vi "Substitute the assigned name for BuildSpecification.vi"(8 "error in":errorcluster, 11 "PluginGenerator_MetaDataObj":refnum<class "PluginGenerator_MetaDataObj.lvclass">) -> (0 "error out":errorcluster, 3 "PluginGenerator_MetaDataObj out":refnum<class "PluginGenerator_MetaDataObj.lvclass">)   [LabVIEW 2023, in "Plugin Generator.lvlib"]
uses:
  Plugin Generator.lvlib
  PluginGenerator_MetaDataObj/PluginGenerator_MetaDataObj.lvclass
  c:/perforce/build/exports/ni/nito/nitoolchainlabview2023eng64/official/export/23.3/23.3.0f52/win/resource/dialog/NewProjectWizard/MetaDataObj/MetaDataObj.lvclass
  <resource>/dialog/NewProjectWizard/MetaDataObj/MetaDataObj.lvclass/MetaDataObj.ctl
  PluginGenerator_MetaDataObj/Accessors/Read User Project Path.vi
  <resource>/dialog/NewProjectWizard/MetaDataObj/Accessors/Read Project Name.vi
  <resource>/dialog/NewProjectWizard/MetaDataObj/Accessors/Read Project Root.vi
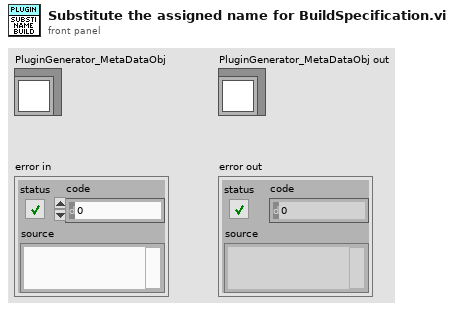
[diagram p1: front panel]
types:
  T1 = enum16{"open", "replace", "create", "open or create", "replace or create", "replace or create with confirmation"}
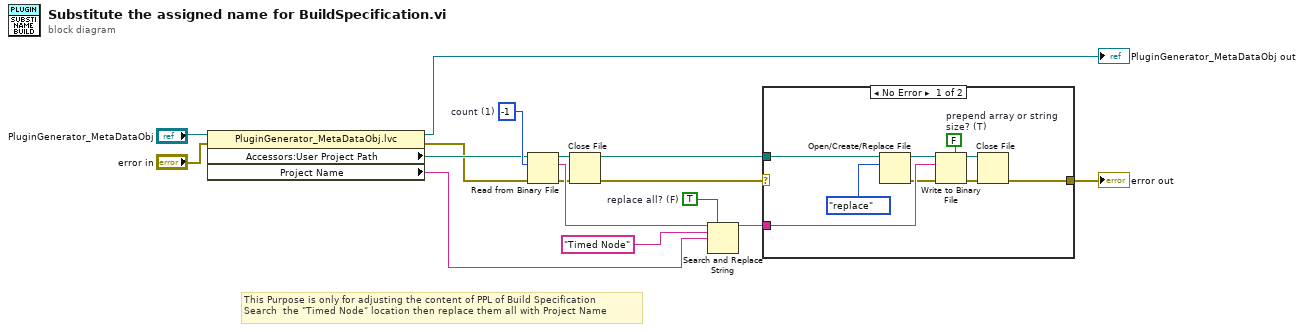
[diagram p0: block diagram]
diagram:
  w13 = TRUE  # replace all? (F)
  w16 = -1  # count (1)
  # "This Purpose is only for adjusting the content of PPL of Build Specification\nSearch  the \"Timed Node\" location then replace them all with Project Name"
  n1 = property class="PluginGenerator_MetaDataObj.lvc"(reference="PluginGenerator_MetaDataObj", error in="error in") -> (reference out=→"PluginGenerator_MetaDataObj out":refnum<class "PluginGenerator_MetaDataObj.lvclass">, error out=w3:errorcluster, "Accessors:User Project Path"=w4:path, "Project Name"=w2:string)
  n2 = Read from Binary File(8:w3, 10:w16, 11:w4) -> (0:w12:errorcluster, 2:w15:string, 3:w11:refnum<file>)  [unwired: 3 in, 1 out]
  n3 = Close File(refnum=w11, error in=w12) -> (path=w8:path, error out=w7:errorcluster)
  n4 = Search and Replace String(replace all?=w13, input string=w15, search string="Timed Node", replace string=w2) -> (result string=w10:string)  [unwired: 4 in, 3 out]
  n5 = case shown="No Error" w7 {
    selector: w7 -> [_ w26]
    tunnel: w10 -> [w23 _]
    tunnel: [w22 w26] -> w9
    tunnel: w8 -> [w20 _]
    frame No Error {
      w17 = FALSE  # prepend array or string size? (T)
      n6 = Open/Create/Replace File(file path (use dialog)=w20, operation (0:open)=T1."replace") -> (refnum out=w18:refnum<file>, error out=w21:errorcluster)  [unwired: 4 in, 1 out]
      n7 = Write to Binary File(file (use dialog)=w18, data=w23, error in=w21, 5:w17) -> (refnum out=w25:refnum<file>, error out=w24:errorcluster)  [unwired: 2 in, 1 out]
      n8 = Close File(refnum=w25, error in=w24) -> (error out=w22:errorcluster)  [unwired: 1 out]
    }
    frame Error {
    }
  }
  "error out" <- w9
